vi "tester.vi"() -> ()   [LabVIEW 2009]
uses:
  <vilib>/Analysis/Matrix/Datatypes/RealMatrix.ctl
  <vilib>/Analysis/Matrix/NI_Matrix.lvlib
panel:
  out "Robot in map":cluster{"Col":dbl, "Row":dbl}
  in  "Walls":cluster{"Col":dbl, "Row":dbl}[](array[cluster])
  in  "Objects bottom cords":T1(array[cluster])
  in  "Robot":cluster{"Col":dbl, "Row":dbl, "Bearing":dbl}
  out "Updated Map":T2
  out "Updated Corners":cluster{"Col":dbl, "Row":dbl}[](array[cluster])
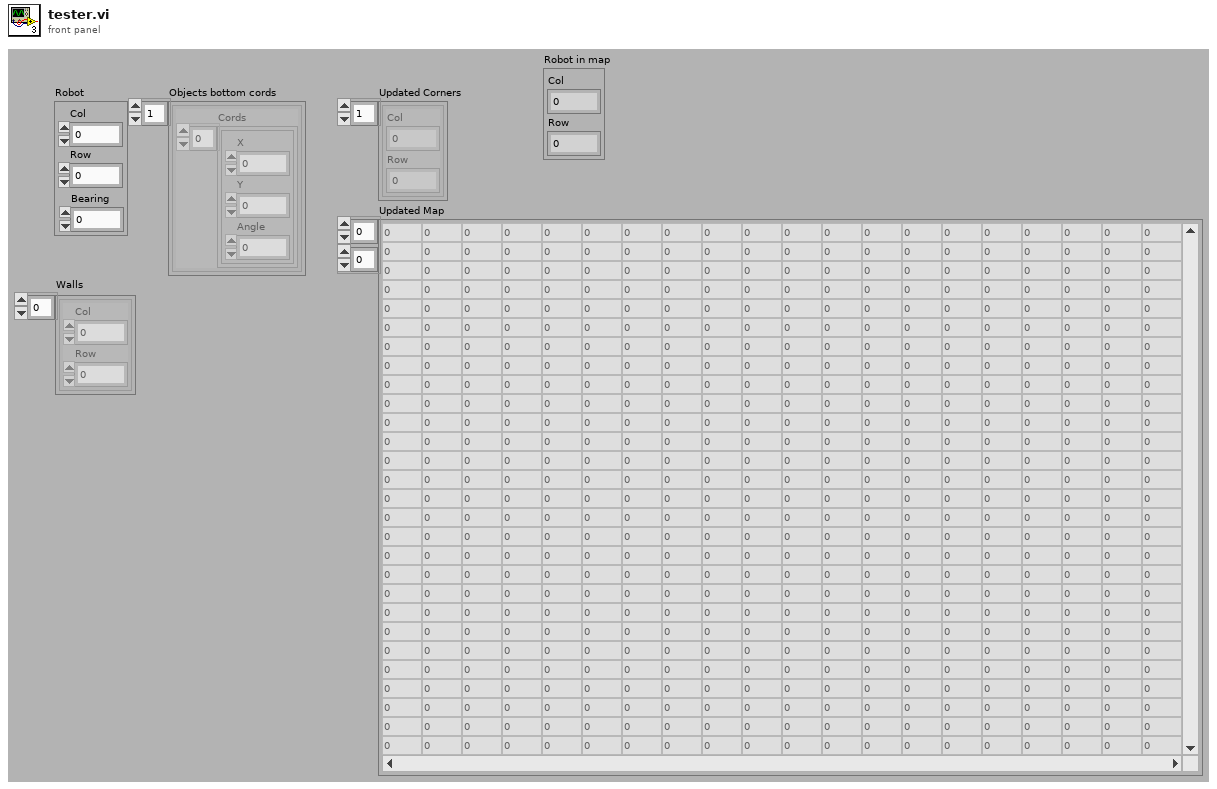
[diagram p1: front panel]
types:
  T1 = cluster{"Cords":cluster{"X":dbl, "Y":dbl, "Angle":dbl}[]}[]
  T2 = typedef "NI_Matrix.lvlib/RealMatrix.ctl" = dbl[][]
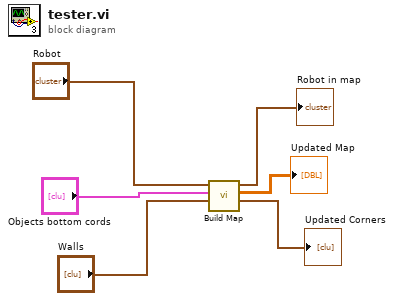
[diagram p0: block diagram]
diagram:
  n1 = call "Build Map.vi"("Walls"="Walls", "Objects bottom cords"="Objects bottom cords", "Robot"="Robot") -> ("Updated Corners"=→"Updated Corners":cluster{"Col":dbl, "Row":dbl}[], "Updated Map"=→"Updated Map":T2, "Robot in map"=→"Robot in map":cluster{"Col":dbl, "Row":dbl})  [unwired: 2 in]
